vi "Testeo_completo_guardado.vi"() -> ()   [LabVIEW 2021]
panel:
  out "error out":errorcluster
  in  "error in (no error)":errorcluster
  out "History Data":T1
  in  "Time Stamp":timestamp
  in  "Nombre":string
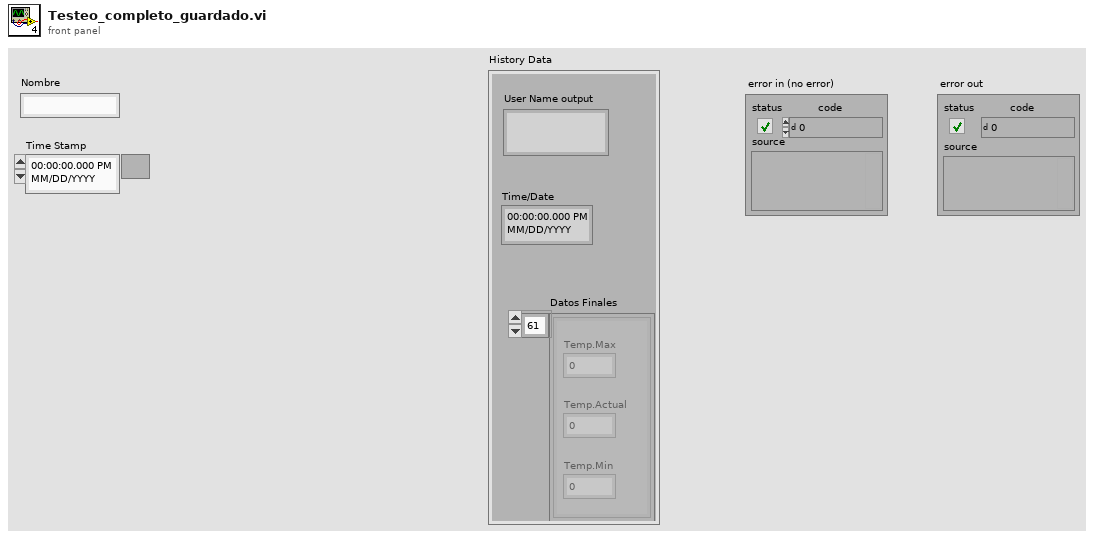
[diagram p1: front panel]
types:
  T1 = cluster{"User Name output":string, "Time/Date":timestamp, "Datos Finales":cluster{"Temp.Max":dbl, "Temp.Actual":dbl, "Temp.Min":dbl}[]}
  T2 = cluster{"Temp.Max":dbl, "Temp.Actual":dbl, "Temp.Min":dbl}[]
  T3 = cluster{"Nombre":string, "Time Stamp ":timestamp, "Datos Finales":cluster{"Temp.Max":dbl, "Temp.Actual":dbl, "Temp.Min":dbl}[]}
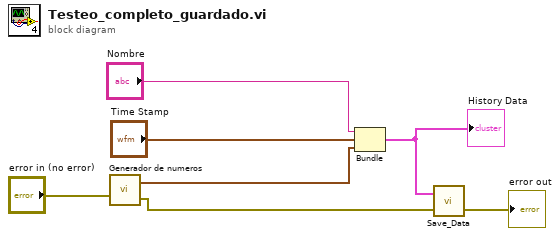
[diagram p0: block diagram]
diagram:
  n1 = call "Generador de numeros.vi"("error in (no error)"="error in (no error)") -> ("error out"=w3:errorcluster, "Datos Finales"=w5:T2)  [unwired: 1 in]
  n2 = Bundle("Nombre"="Nombre", "Time Stamp"="Time Stamp", "Datos Finales"=w5) -> (w2:T3)  [unwired: 1 in]
  "History Data" <- w2
  n3 = call "Save_Data.vi"("error in (no error)"=w3, "History Data"=w2) -> ("error out"=→"error out":errorcluster)  [unwired: 1 in]
